vi "Probe tip Calibration Check.vi"() -> ()   [LabVIEW 2020]
uses:
  <vilib>/addons/HF Network Analysis/Support VIs/Read SnP File (SnP).vi
  <vilib>/addons/HF Network Analysis/NI_HFNetworkAnalysis.lvlib
  <vilib>/Analysis/NI_AALPro.lvlib
panel:
  out "Short Resistance":cluster{dbl[], dbl[]}[](graph)
  in  "Thru":path
  out "Thru delay":cluster{"Frequencies (Hz)":dbl[], dbl[]}(graph)
  in  "Short":path
  out "Short Inductance":cluster{dbl[], dbl[]}[](graph)
  out "Open capacitance":cluster{dbl[], dbl[]}[](graph)
  in  "Open":path
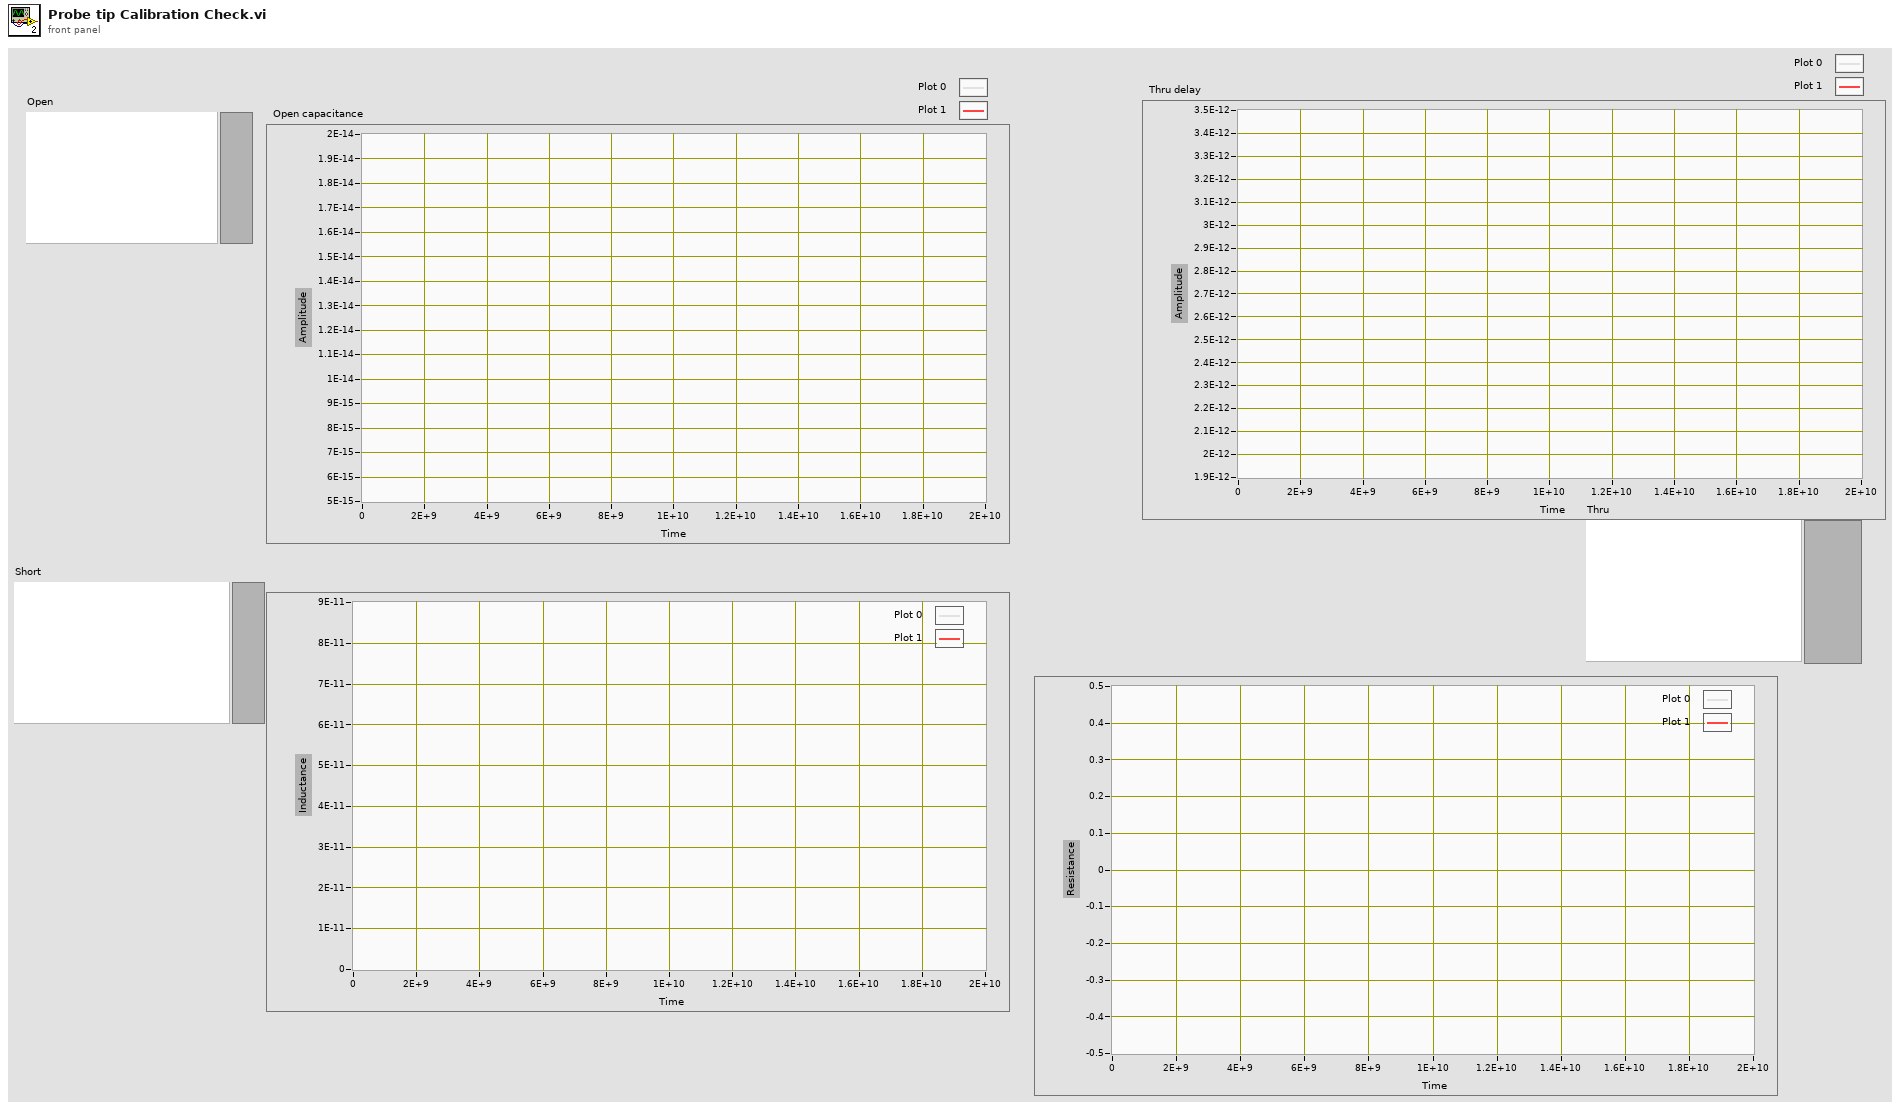
[diagram p1: front panel]
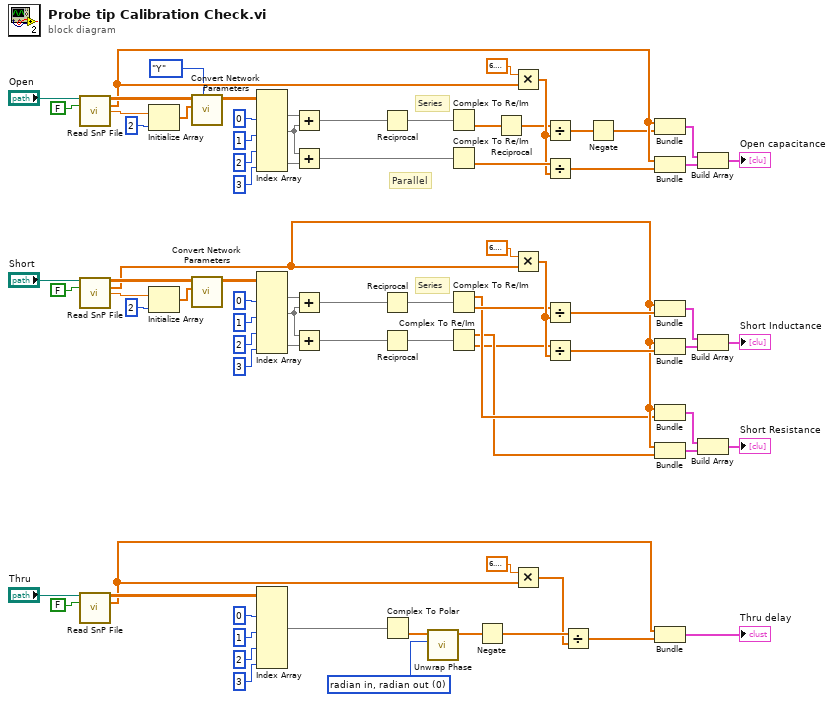
[diagram p0: block diagram]
diagram:
  w10 = 0 items=["radian in, radian out", "radian in, degree out", "degree in, degree out", "degree in, radian out"] ("phase unit")
  # "Series"
  # "Series"
  # "Parallel"
  n1 = call-poly <vilib>:"Read SnP File.vi"("SnP File Path"="Open", "Swap Ports (False)"=FALSE) -> ("S-parameters"=w78:cdb[][], "Frequencies (Hz)"=w38:dbl[], "Z0 (Ohm)"=w77:cdb)  [unwired: 10 in, 1 out]
  n2 = call-poly <vilib>:"Read SnP File.vi"("SnP File Path"="Short", "Swap Ports (False)"=FALSE) -> ("S-parameters"=w41:cdb[][], "Frequencies (Hz)"=w6:dbl[], "Z0 (Ohm)"=w42:cdb)  [unwired: 10 in, 1 out]
  n3 = call-poly <vilib>:"Read SnP File.vi"("SnP File Path"="Thru", "Swap Ports (False)"=FALSE) -> ("S-parameters"=w20:cdb[][], "Frequencies (Hz)"=w14:dbl[])  [unwired: 10 in, 2 out]
  n4 = Initialize Array(w77, 2 ("dimension size")) -> (w76:cdb[])
  n5 = Initialize Array(w42, 2 ("dimension size")) -> (w43:cdb[])
  n6 = call "Convert Network Parameters.vi"("Parameters to convert"=enum16{"Y", "Z", "T"}."Y", "Zc (Ohm)"=w76, "S-par Array In"=w78) -> ("Y/Z Array Out"=w68:cdb[][])  [unwired: 6 in, 2 out]
  n7 = call "Convert Network Parameters.vi"("Zc (Ohm)"=w43, "S-par Array In"=w41) -> ("Y/Z Array Out"=w50:cdb[][])  [unwired: 7 in, 2 out]
  n8 = Index Array(array=w68, index (col) #1=0 ("disabled index (col)"), index (col) #2=1 ("disabled index (col)"), index (col) #3=2 ("index (col)"), index (col) #4=3 ("index (col)")) -> (element #1=w70:cdb[], element #2=w67:cdb[], element #4=w66:cdb[])  [unwired: 4 in, 1 out]
  n9 = Index Array(array=w50, index (col) #1=0 ("disabled index (col)"), index (col) #2=1 ("disabled index (col)"), index (col) #3=2 ("index (col)"), index (col) #4=3 ("index (col)")) -> (element #1=w49:cdb[], element #2=w51:cdb[], element #4=w52:cdb[])  [unwired: 4 in, 1 out]
  n10 = Index Array(array=w20, index (col) #1=0 ("disabled index (col)"), index (col) #2=1 ("disabled index (col)"), index (col) #3=2 ("index (col)"), index (col) #4=3 ("index (col)")) -> (element #2=w19:cdb[])  [unwired: 4 in, 3 out]
  n11 = Add(x=w70, y=w67) -> (x+y=w36:cdb[])
  n12 = Add(x=w67, y=w66) -> (x+y=w65:cdb[])
  n13 = Add(x=w49, y=w51) -> (x+y=w30:cdb[])
  n14 = Add(x=w51, y=w52) -> (x+y=w2:cdb[])
  n15 = Reciprocal(x=w36) -> (1/x=w35:cdb[])
  n16 = Reciprocal(x=w30) -> (1/x=w29:cdb[])
  n17 = Reciprocal(x=w2) -> (1/x=w1:cdb[])
  n18 = Complex To Polar(r * e^(i*theta)=w19) -> (theta=w12:dbl[])  [unwired: 1 out]
  n19 = call <vilib>:"Unwrap Phase.vi"("phase unit"=w10, "Phase"=w12) -> ("Unwrapped Phase"=w11:dbl[])  [unwired: 8 in, 1 out]
  n20 = Complex To Re/Im(x + iy=w35) -> (y=w34:dbl[])  [unwired: 1 out]
  n21 = Complex To Re/Im(x + iy=w65) -> (y=w69:dbl[])  [unwired: 1 out]
  n22 = Complex To Re/Im(x + iy=w29) -> (x=w5:dbl[], y=w27:dbl[])
  n23 = Complex To Re/Im(x + iy=w1) -> (x=w4:dbl[], y=w3:dbl[])
  n24 = Negate(x=w11) -> (-x=w16:dbl[])
  n25 = Reciprocal(x=w34) -> (1/x=w33:dbl[])
  n26 = Multiply(x=6.283185307179586, y=w38) -> (x*y=w62:dbl[])
  n27 = Multiply(x=6.283185307179586, y=w6) -> (x*y=w55:dbl[])
  n28 = Multiply(x=6.283185307179586, y=w14) -> (x*y=w13:dbl[])
  n29 = Divide(x=w33, y=w62) -> (x/y=w32:dbl[])
  n30 = Divide(x=w69, y=w62) -> (x/y=w63:dbl[])
  n31 = Divide(x=w27, y=w55) -> (x/y=w54:dbl[])
  n32 = Divide(x=w3, y=w55) -> (x/y=w28:dbl[])
  n33 = Divide(x=w16, y=w13) -> (x/y=w18:dbl[])
  n34 = Negate(x=w32) -> (-x=w31:dbl[])
  n35 = Bundle("Frequencies (Hz)"=w38, w31) -> (w61:cluster{"Frequencies (Hz)":dbl[], dbl[]})  [unwired: 1 in]
  n36 = Bundle("Frequencies (Hz)"=w38, w63) -> (w60:cluster{"Frequencies (Hz)":dbl[], dbl[]})  [unwired: 1 in]
  n37 = Bundle("Frequencies (Hz)"=w6, w54) -> (w56:cluster{"Frequencies (Hz)":dbl[], dbl[]})  [unwired: 1 in]
  n38 = Bundle("Frequencies (Hz)"=w6, w28) -> (w57:cluster{"Frequencies (Hz)":dbl[], dbl[]})  [unwired: 1 in]
  n39 = Bundle("Frequencies (Hz)"=w6, w5) -> (w9:cluster{"Frequencies (Hz)":dbl[], dbl[]})  [unwired: 1 in]
  n40 = Bundle("Frequencies (Hz)"=w6, w4) -> (w8:cluster{"Frequencies (Hz)":dbl[], dbl[]})  [unwired: 1 in]
  n41 = Bundle("Frequencies (Hz)"=w14, w18) -> (→"Thru delay":cluster{"Frequencies (Hz)":dbl[], dbl[]})  [unwired: 1 in]
  n42 = Build Array(w61, w60) -> (→"Open capacitance":cluster{"Frequencies (Hz)":dbl[], dbl[]}[])
  n43 = Build Array(w56, w57) -> (→"Short Inductance":cluster{"Frequencies (Hz)":dbl[], dbl[]}[])
  n44 = Build Array(w9, w8) -> (→"Short Resistance":cluster{"Frequencies (Hz)":dbl[], dbl[]}[])
